vi "initializeLED.vi"(8 "error in (no error)":errorcluster, 9 "frequency":dbl=10.0 format="%0.2p", 10 "LED Refnum":refnum<vi>) -> (0 "error out":errorcluster, 3 "LED out":refnum<class "LED.lvclass">)   [LabVIEW 2019, in "LED.lvclass"]
doc: "connects the UI LED Controller to the class through its reference."
uses:
  LED.lvclass
  LED.lvclass/LED.ctl
  Sound/Sound.lvclass
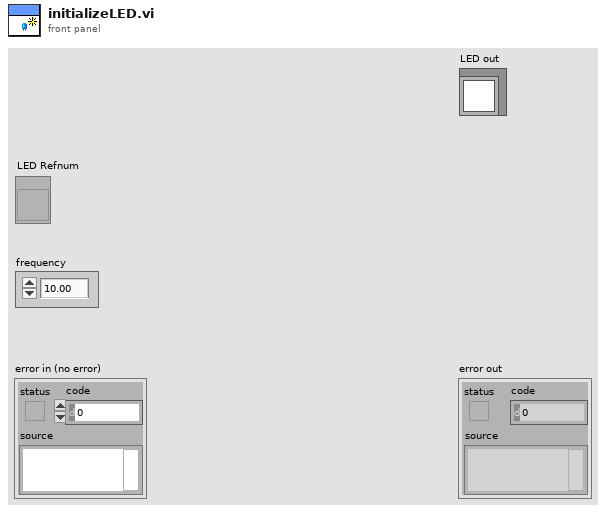
[diagram p1: front panel]
types:
  T1 = cluster{"Device ID":u32, "Volume":dbl, "frequency":dbl, "duration (s)":dbl}
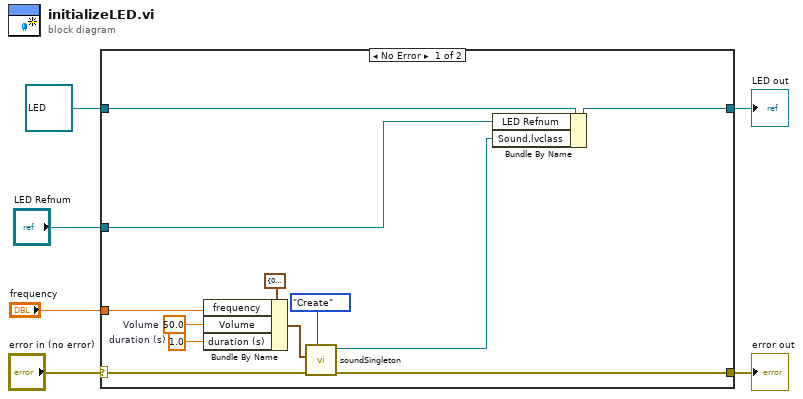
[diagram p0: block diagram]
diagram:
  n1 = case shown="No Error" "error in (no error)" {
    selector: "error in (no error)" -> [w17 w20]
    tunnel: [w14 w20] -> w5
    tunnel: [w16 w19] -> w3
    tunnel: refnum<class "LED.lvclass"> refnum ("LED in") -> [w18 w19]
    tunnel: "LED Refnum" -> [w15 _]
    tunnel: "frequency" -> [w10 _]
    frame No Error {
      w9 = 50.0  # Volume
      w8 = 1.0  # duration (s)
      n2 = Bundle By Name(cluster=T1 {"Device ID"=0, "Volume"=50.0, "frequency"=10.0, "duration (s)"=0.0} ("Sound Parameters"), "frequency"=w10, "Volume"=w9, "duration (s)"=w8) -> (w11:T1)
      n3 = call "soundSingleton.vi"("Option"=enum16{"Create", "Destroy"}."Create", "error in (no error)"=w17, "Sound Parameters"=w11) -> ("error out"=w14:errorcluster, "Sound out"=w13:refnum<class "Sound.lvclass">)  [unwired: 7 in]
      n4 = Bundle By Name(cluster=w18, "LED Refnum"=w15, "Sound.lvclass"=w13) -> (w16:refnum<class "LED.lvclass">)
    }
    frame Error {
    }
  }
  "error out" <- w5
  "LED out" <- w3
